vi "StartServer.vi"(8 "error in (no error)":errorcluster, 11 "Server in":refnum<class "Server.lvclass">) -> (0 "error out":errorcluster, 3 "Server out":refnum<class "Server.lvclass">)   [LabVIEW 2017, in "opcua.lvlib" / "Server.lvclass"]
uses:
  Server.lvclass
  Server.lvclass/Server.ctl
  opcua32.dll
  opcua.lvlib
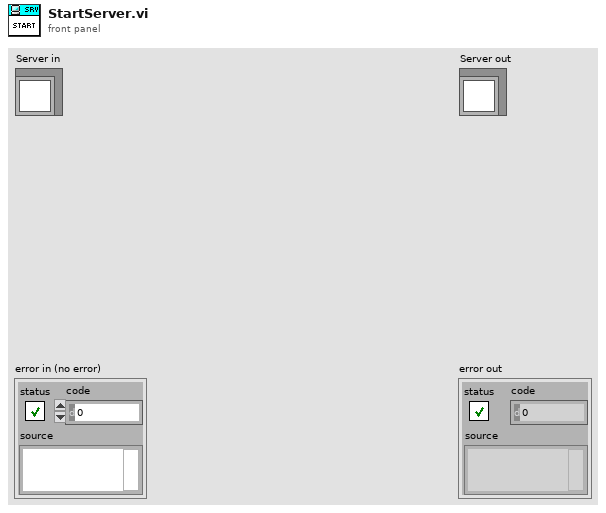
[diagram p1: front panel]
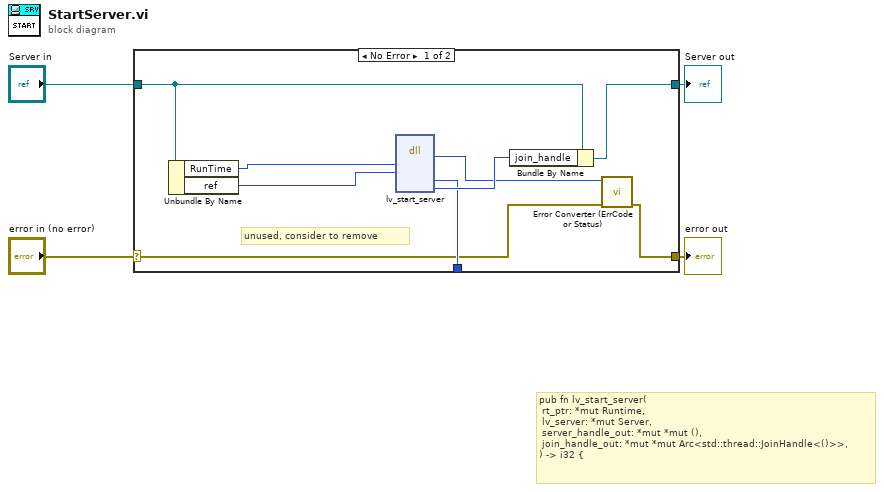
[diagram p0: block diagram]
diagram:
  # "pub fn lv_start_server(\n\trt_ptr: *mut Runtime,\n\tlv_server: *mut Server,\n\tserver_handle_out: *mut *mut (),\n\tjoin_handle_out: *mut *mut Arc<std::thread::JoinHandle<()>>,\n) -> i32 {"
  n1 = case shown="No Error" "error in (no error)" {
    selector: "error in (no error)" -> [w7 w14]
    tunnel: [w6 w14] -> w3
    tunnel: [w10 w15] -> w1
    tunnel: "Server in" -> [w11 w15]
    tunnel: [w8 _] -> _
    frame No Error {
      # "unused, consider to remove"
      n2 = Unbundle By Name(w11) -> ("RunTime"=w13:u64, "ref"=w12:u64)
      n3 = dll-call lib="C:/Users/Andrey/Desktop/opcua-labview/opcua-lvlib/opcua*.dll" fn="lv_start_server"("RunTime"=w13, "server_ref"=w12) -> ("return type"=w5:i32, "server_handle_out"=w8:u64, "join_handle_out"=w9:u64)  [unwired: 7 in, 2 out]
      n4 = Bundle By Name(cluster=w11, "join_handle"=w9) -> (w10:refnum<class "Server.lvclass">)
      n5 = call "Error Converter (ErrCode or Status).vi"("error in (no error)"=w7, "error code"=w5) -> ("error out"=w6:errorcluster)  [unwired: 9 in]
    }
    frame Error {
    }
  }
  "error out" <- w3
  "Server out" <- w1
